vi "ExcitationParameters_v2.vi"(6 "heartBeatSimParams":T1={"curveParams"={"amplitude"=0.2, "peakHeight"=0.05, "cycleLength"=0, "snapIn"=0.001, "adhesion"=0.02, "peakShift"=0, "noiseAmplitude"=0.0001, "asymmetry"=0.1}, "cantileverParams"={"samplingRate"=1000000.0, "cantileverFreq"=500000.0, "qFactor"=2.0}} {"cantileverParams"."cantileverFreq" format="%#_6p"; "cantileverParams"."samplingRate" format="%#_6p"}, 7 "outputRange":dbl=1.0, 8 "error in":errorcluster, 9 "excitationParameters":T3 {"shift" min=-1.0 max=1.0}, 10 "ioFreqHz":u32, 11 "FPGA VI Reference In":T2) -> (0 "error out":errorcluster, 2 "WaveSize":i32, 3 "FPGA VI Reference Out":T2, 4 "Excitation":dbl[](array[numeric]))   [LabVIEW 2016]
uses:
  controls/FPGAVIreferenceTypeDef.ctl
  controls/Enum.ctl
  <vilib>/Utility/error.llb/Error Cluster From Error Code.vi
  <vilib>/rvi/errors/niLvFpgaAdjustHostInterfaceError.vi
  <vilib>/rvi/interface/nirviReadWriteControl/nirviReadWriteControl.xnode
  FPGA Bitfiles/qnmController797_usbRIO_controllerFPGAmu.lvbitx
  NiFpgaLv.dll
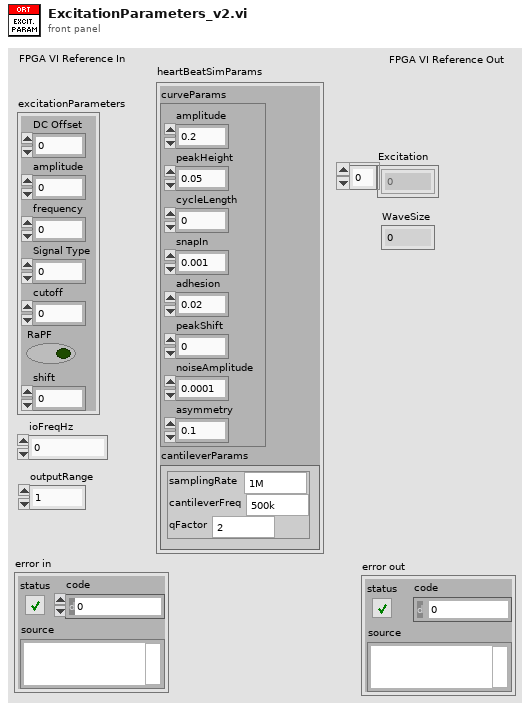
[diagram p1: front panel]
types:
  T1 = cluster{"curveParams":cluster{"amplitude":dbl, "peakHeight":dbl, "cycleLength":u16, "snapIn":dbl, "adhesion":dbl, "peakShift":u16, "noiseAmplitude":dbl, "asymmetry":dbl}, "cantileverParams":cluster{"samplingRate":dbl, "cantileverFreq":dbl, "qFactor":dbl}}
  T2 = typedef "FPGAVIreferenceTypeDef.ctl" = refnum<k20>
  T3 = cluster{"DC Offset":dbl, "amplitude":dbl, "frequency":dbl, "Signal Type":u16, "cutoff":dbl, "RaPF":bool, "shift":dbl}
  T4 = typedef "Enum.ctl" = enum16{"Init", "Read", "Write"}
  T5 = cluster{"scanEngineHz":u32, "feedbackHz":u32, "sicmHz":u32, "rampHz":u32}
  T6 = cluster{"amplitude":dbl, "peakHeight":dbl, "cycleLength":u16, "snapIn":dbl, "adhesion":dbl, "peakShift":u16, "noiseAmplitude":dbl, "asymmetry":dbl}
  T7 = cluster{"samplingRate":dbl, "cantileverFreq":dbl, "qFactor":dbl}
  T8 = cluster{"maxLoc":u16, "threshold":i16, "fitHardPtLimit":u16}
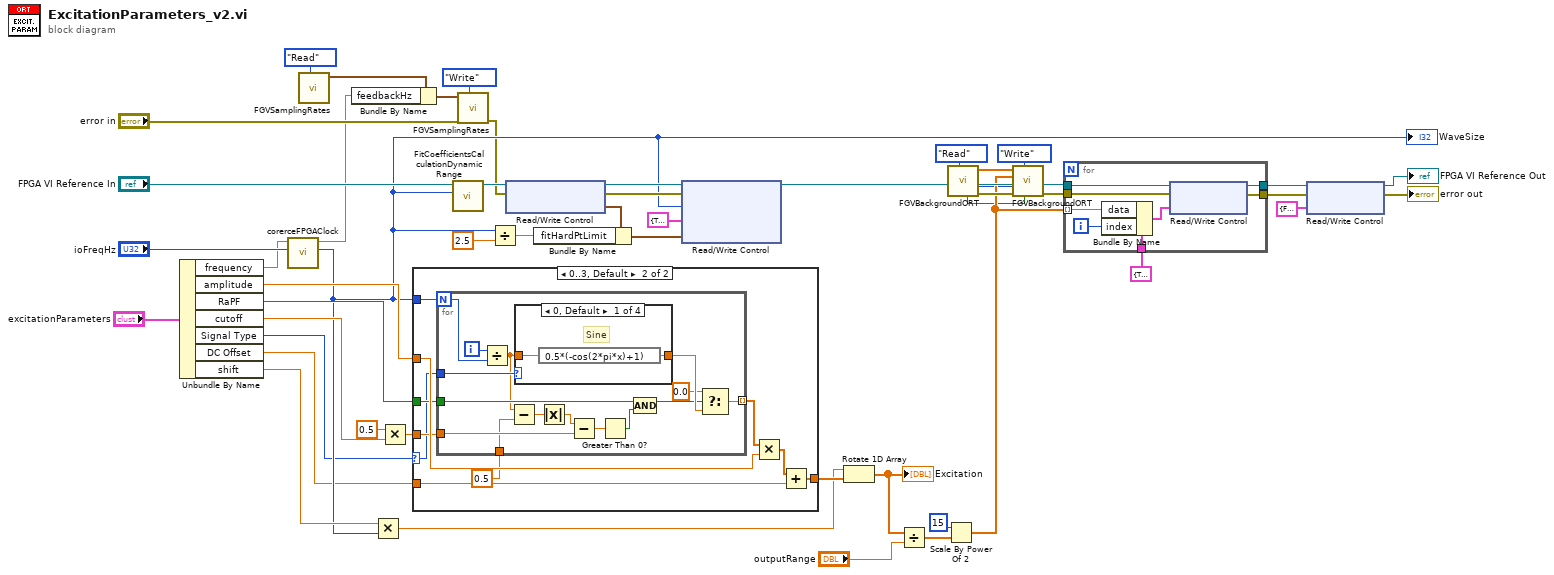
[diagram p0: block diagram]
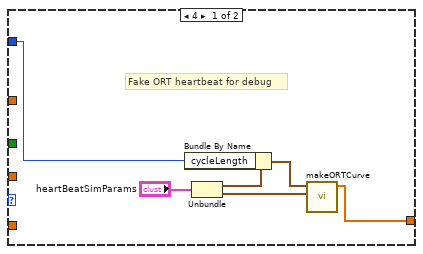
[diagram p2: hidden frame]
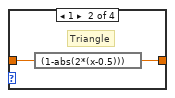
[diagram p3: hidden frame]
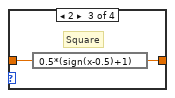
[diagram p4: hidden frame]
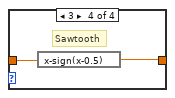
[diagram p5: hidden frame]
diagram:
  n1 = Unbundle By Name("excitationParameters") -> ("frequency"=w5:dbl, "amplitude"=w44:dbl, "RaPF"=w43:bool, "cutoff"=w42:dbl, "Signal Type"=w3:u16, "DC Offset"=w4:dbl, "shift"=w33:dbl)
  n2 = call "corerceFPGAClock.vi"("baseClock"="ioFreqHz", "requestedFrequency"=w5) -> ("decimation"=w10:u16, "realFrequency"=w7:dbl)  [unwired: 7 in, 1 out]
  "WaveSize" <- w10
  n3 = call "FGVSamplingRates.vi"("Enum"=Enum."Read") -> ("samplingRatesOut"=w12:T5)  [unwired: 9 in, 1 out]
  n4 = Bundle By Name(cluster=w12, "feedbackHz"=w7) -> (w11:T5)
  n5 = Multiply(x=w33, y=w10) -> (x*y=w32:dbl)
  n6 = Multiply(x=0.5, y=w42) -> (x*y=w38:dbl)
  n7 = case shown="0..3, Default" w3 {
    selector: w3 -> [_ w57]
    tunnel: w10 -> [w50 w65]
    tunnel: w4 -> [_ w64]
    tunnel: [w55 w63] -> w35
    tunnel: w44 -> [_ w60]
    tunnel: w43 -> [_ w59]
    tunnel: w38 -> [_ w58]
    frame 4 {
      # "Fake ORT heartbeat for debug"
      n8 = Unbundle("heartBeatSimParams") -> ("curveParams"=w52:T6, "cantileverParams"=w53:T7)
      n9 = Bundle By Name(cluster=w52, "cycleLength"=w50) -> (w51:T6)
      n10 = call "makeORTCurve.vi"("cantileverParams"=w53, "curveParams"=w51) -> ("ortCurve"=w55:dbl[])  [unwired: 9 in]
    }
    frame 0..3, Default {
      n11 = for {
        N: w65 -> [w78]
        tunnel: w57 -> [w80]
        tunnel: [w76] -> w62 mode=indexing
        tunnel: w59 -> [w77]
        tunnel: w58 -> [w70]
        tunnel: 0.5 ("y") -> [w66]
        i -> [w79]
        n12 = Divide(x=w79, y=w78) -> (x/y=w73:dbl)
        n13 = Subtract(x=w73, y=w66) -> (x-y=w72:dbl)
        n14 = case shown="0, Default" w80 {
          tunnel: w73 -> [w82 w84 w85 w88]
          tunnel: [w81 w83 w86 w87] -> w75
          frame 0, Default {
            # "Sine"
            n15 = expression code="0.5*(-cos(2*pi*x)+1)"(w82) -> (w81:dbl)
          }
          frame 1 {
            # "Triangle"
            n16 = expression code="(1-abs(2*(x-0.5)))"(w84) -> (w83:dbl)
          }
          frame 2 {
            # "Square"
            n17 = expression code="0.5*(sign(x-0.5)+1)"(w85) -> (w86:dbl)
          }
          frame 3 {
            # "Sawtooth"
            n18 = expression code="x-sign(x-0.5)"(w88) -> (w87:dbl)
          }
        }
        n19 = Absolute Value(x=w72) -> (abs(x)=w71:dbl)
        n20 = Subtract(x=w71, y=w70) -> (x-y=w69:dbl)
        n21 = Greater Than 0?(x=w69) -> (x > 0?=w68:bool)
        n22 = Compound Arithmetic op=AND(w77, w68) -> (w74:bool)
        n23 = Select(t=0.0, s=w74, f=w75) -> (s? t:f=w76:dbl)
      }
      n24 = Multiply(x=w62, y=w60) -> (x*y=w61:dbl[])
      n25 = Add(x=w61, y=w64) -> (x+y=w63:dbl[])
    }
  }
  n26 = call "FitCoefficientsCalculationDynamicRange.vi"("ArraySize"=w10, "FPGA VI Reference In"="FPGA VI Reference In") -> ("FPGA VI Reference Out"=w26:T2)  [unwired: 9 in]
  n27 = call "FGVSamplingRates.vi"("Enum"=Enum."Write", "error in"="error in", "samplingRatesIn"=w11) -> ("error out"=w8:errorcluster)  [unwired: 7 in, 1 out]
  n28 = Divide(x=w10, y=2.5) -> (x/y=w31:dbl)
  n29 = xnode "Read/Write Control"("FPGA VI Reference In"=w26, "error in"=w8) -> ("FPGA VI Reference Out"=w17:T2, "error out"=w16:errorcluster, "ort.fit.p.params"=w25:T8)
  n30 = Bundle By Name(cluster=w25, "fitHardPtLimit"=w31) -> (w18:T8)
  n31 = xnode "Read/Write Control"("FPGA VI Reference In"=w17, "error in"=w16, "ort.p.waveSize"=w10, "aio.m.drive"=cluster{"write":bool, "data":i16, "index":u16} {"write"=TRUE, "data"=0, "index"=0} ("outWaveWrite"), "ort.fit.p.params"=w18) -> ("FPGA VI Reference Out"=w48:T2)  [unwired: 1 out]
  n32 = Rotate 1D Array(1:w35, 2:w32) -> (0:w34:dbl[])
  "Excitation" <- w34
  n33 = Divide(x=w34, y="outputRange") -> (x/y=w41:dbl[])
  n34 = Scale By Power Of 2(n=i16 15, x=w41) -> (x*2^n=w39:dbl[])
  n35 = call "FGVBackgroundORT.vi"("Enum"=Enum."Read") -> ("error out"=w47:errorcluster, "arrayOut"=w27:i16[], "Wave Out Shifted"=w1:dbl[], "Corrected...Out"=w2:bool)  [unwired: 6 in, 1 out]
  n36 = call "FGVBackgroundORT.vi"("Corrected...In"=w2, "Enum"=Enum."Write", "error in"=w47, "arrayIn"=w27, "Wave In"=w39, "Wave In Shifted"=w1) -> ("error out"=w15:errorcluster)  [unwired: 1 in, 4 out]
  n37 = for {
    tunnel: w39 -> [w95] mode=indexing
    tunnel: w48 -> [w94]
    tunnel: [w92] -> w22
    tunnel: w15 -> [w91]
    tunnel: [w90] -> w23
    tunnel: cluster{"write":bool, "data":i16, "index":u16} {"write"=TRUE, "data"=0, "index"=0} ("outWaveWrite") -> [w89]
    i -> [w96]
    n38 = Bundle By Name(cluster=w89, "data"=w95, "index"=w96) -> (w93:cluster{"write":bool, "data":i16, "index":u16})
    n39 = xnode "Read/Write Control"("FPGA VI Reference In"=w94, "error in"=w91, "aio.m.drive"=w93) -> ("FPGA VI Reference Out"=w92:T2, "error out"=w90:errorcluster)
  }
  n40 = xnode "Read/Write Control"("FPGA VI Reference In"=w22, "error in"=w23, "aio.m.drive"=cluster{"write":bool, "data":i16, "index":u16} {"write"=FALSE, "data"=0, "index"=0} ("outWaveWrite")) -> ("FPGA VI Reference Out"=→"FPGA VI Reference Out":T2, "error out"=→"error out":errorcluster)
